vi "Global texto reporte.vi"() -> ()   [LabVIEW 2009]
panel:
  in  "Partial Report":string
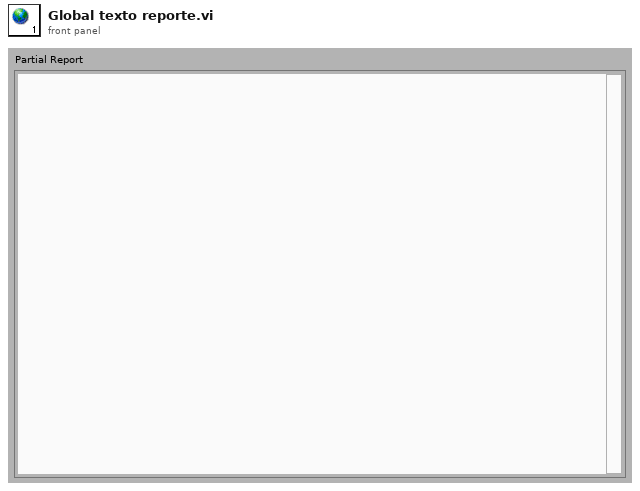
[diagram p1: front panel]
diagram:
